vi "lijnvolgen afstandssensor.vi"() -> ()   [LabVIEW 2019]
uses:
  <vilib>/myRIO/Common/Instrument Driver Framework/Utilities/typedefs/Analog Scaling Constants.ctl
  <vilib>/myRIO/Common/Instrument Driver Framework/Utilities/typedefs/Analog Scaling Constants List.ctl
  <vilib>/myRIO/Common/Instrument Driver Framework/myRIO v1.0/AO/typedefs/AO Channels Enum.ctl
  <vilib>/myRIO/Common/Instrument Driver Framework/myRIO v1.0/AO/typedefs/AO Channels List.ctl
  <vilib>/myRIO/Common/Instrument Driver Framework/Utilities/typedefs/Generic FPGA Reference.ctl
  <vilib>/myRIO/Common/Instrument Driver Framework/Utilities/typedefs/myRIO v1.0 Reference.ctl
  <vilib>/myRIO/Common/Instrument Driver Framework/Utilities/typedefs/Hardware Version Enum.ctl
  <vilib>/myRIO/Common/Instrument Driver Framework/Utilities/typedefs/myRIO Generic Hardware Reference.ctl
  <vilib>/myRIO/Instrument Drivers/Onboard IO/AO/typedefs/AO Reference.ctl
  <vilib>/myRIO/Instrument Drivers/Onboard IO/AO/AO.lvlib
  <vilib>/myRIO/Instrument Drivers/Onboard IO/AO/vis/Write.vi
  <vilib>/userDefined/High Color/nirio_resource_hc.ctl
  <vilib>/myRIO/Common/Instrument Driver Framework/myRIO v1.0/AO/vis/myRIO v1.1 Open AO.vi
  <vilib>/myRIO/Instrument Drivers/Onboard IO/AO/vis/myRIO AO Open.xnode
  <vilib>/myRIO/Common/Instrument Driver Framework/Utilities/vis/Is FPGA Ref Available.vi
  <vilib>/myRIO/Express VI/Onboard IO/AO/AO Express VI.xnode
  <vilib>/myRIO/Common/Instrument Driver Framework/myRIO v1.0/AI/typedefs/AI Channels Enum.ctl
  <vilib>/myRIO/Common/Instrument Driver Framework/myRIO v1.0/AI/typedefs/AI Channels List.ctl
  <vilib>/myRIO/Instrument Drivers/Onboard IO/AI/typedefs/AI Reference.ctl
  <vilib>/myRIO/Instrument Drivers/Onboard IO/AI/AI.lvlib
  <vilib>/myRIO/Instrument Drivers/Onboard IO/AI/vis/Read.vi
  <vilib>/myRIO/Common/Instrument Driver Framework/myRIO v1.0/AI/vis/myRIO v1.1 Open AI.vi
  <vilib>/myRIO/Instrument Drivers/Onboard IO/AI/vis/myRIO AI Open.xnode
  <vilib>/myRIO/Express VI/Onboard IO/AI/AI Express VI.xnode
  <vilib>/myRIO/Common/Instrument Driver Framework/myRIO v1.0/DIO/typedefs/DIO Channels Enum.ctl
  <vilib>/myRIO/Common/Instrument Driver Framework/myRIO v1.0/DIO/typedefs/DIO Channels List.ctl
  <vilib>/myRIO/Instrument Drivers/Onboard IO/DIO/typedefs/DIO Reference.ctl
  <vilib>/myRIO/Instrument Drivers/Onboard IO/DIO/DIO.lvlib
  <vilib>/myRIO/Instrument Drivers/Onboard IO/DIO/vis/Read.vi
  <vilib>/myRIO/Common/Instrument Driver Framework/myRIO v1.0/DIO/vis/myRIO v1.1 Open DIO.vi
  <vilib>/myRIO/Instrument Drivers/Onboard IO/DIO/vis/myRIO DIO Open.xnode
  <vilib>/myRIO/Express VI/Onboard IO/DI/DI Express VI.xnode
panel:
  out "GEEN obstakel":bool
  in  "Hoofdwhile":bool
  out "Numeric 4":i32
  out "analoog":dbl[](array[numeric])
  out "Array 3":i32[](array[numeric])
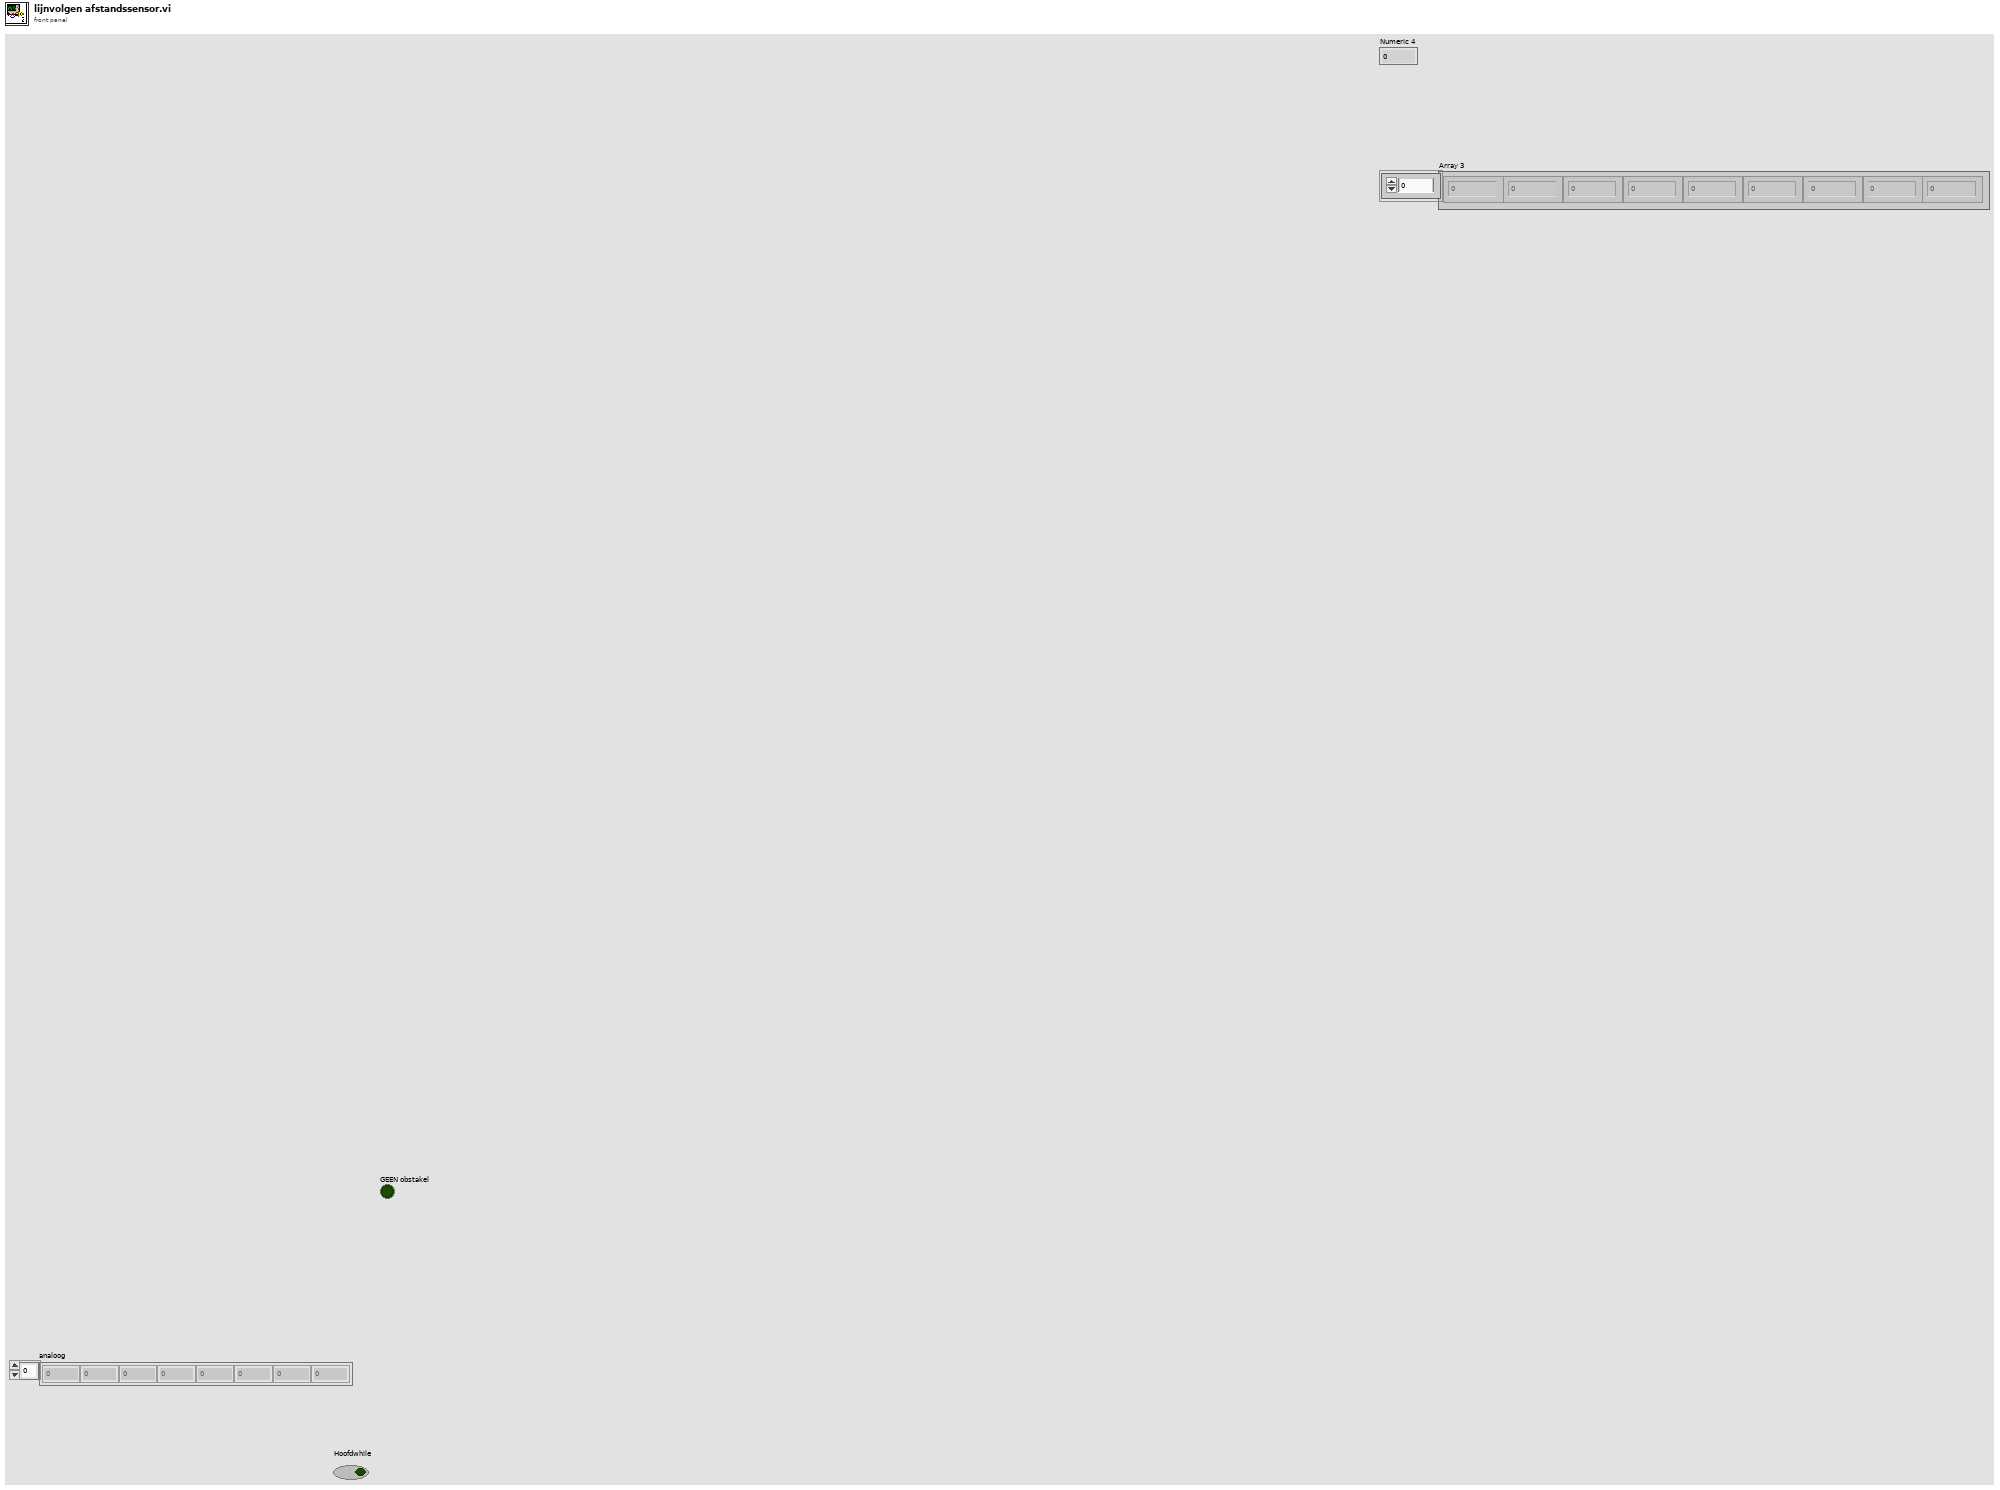
[diagram p1: front panel]
types:
  T1 = typedef "AO.lvlib/AO Reference.ctl" = cluster{"myRIO Reference":T2, "AO Channel List":T6, "AO Scaling Constant List":T8}
  T2 = typedef "myRIO Generic Hardware Reference.ctl" = cluster{"myRIO Model":T3, "myRIO Hardware Reference":T4}
  T3 = typedef "Hardware Version Enum.ctl" = enum16{"Unknown", "myRIO-1900", "myRIO-1950", "roboRIO", "NI ELVIS RIO CM", "ELVIS III"}
  T4 = typedef "myRIO v1.0 Reference.ctl" = cluster{"Generic FPGA Reference":T5, "Allow multiple opens":bool}
  T5 = typedef "Generic FPGA Reference.ctl" = refnum<k20>
  T6 = typedef "AO Channels List.ctl" = T7[]
  T7 = typedef "AO Channels Enum.ctl" = enum16{"Not Connected", "AudioOut/Left", "AudioOut/Right", "C/AO0", "C/AO1", "A/AO0", "A/AO1", "B/AO0", "B/AO1"}
  T8 = typedef "Analog Scaling Constants List.ctl" = T9[]
  T9 = typedef "Analog Scaling Constants.ctl" = cluster{"LSB Weight (Volts)":dbl, "Offset (Volts)":dbl, "Signed?":bool}
  T10 = typedef "nirio_resource_hc.ctl" = tag
  T11 = typedef "AI.lvlib/AI Reference.ctl" = cluster{"myRIO Reference":T2, "AI Channels List":T12, "AI Scaling Constants List":T8}
  T12 = typedef "AI Channels List.ctl" = T13[]
  T13 = typedef "AI Channels Enum.ctl" = enum16{"Not Connected", "AudioIn/Left", "AudioIn/Right", "C/AI0", "C/AI1", "A/AI0", "A/AI1", "A/AI2", "A/AI3", "A/AI4", "A/AI5", "A/AI6", "A/AI7", "B/AI0", "B/AI1", "B/AI2", "B/AI3", "B/AI4", "B/AI5", "B/AI6", "B/AI7", "AI/AI0", "AI/AI1", "AI/AI2", "AI/AI3", "A/AI0 (DIFF)", "A/AI1 (DIFF)", "A/AI2 (DIFF)", "A/AI3 (DIFF)", "B/AI0 (DIFF)", "B/AI1 (DIFF)", "B/AI2 (DIFF)", "B/AI3 (DIFF)"}
  T14 = typedef "DIO.lvlib/DIO Reference.ctl" = cluster{"myRIO Reference":T2, "DIO Channels List":T15}
  T15 = typedef "DIO Channels List.ctl" = T16[]
  T16 = typedef "DIO Channels Enum.ctl" = enum16{"Not Connected", "C/DIO0", "C/DIO1", "C/DIO2", "C/DIO3", "C/DIO4", "C/DIO5", "C/DIO6", "C/DIO7", "A/DIO0", "A/DIO1", "A/DIO2", "A/DIO3", "A/DIO4", "A/DIO5", "A/DIO6", "A/DIO7", "A/DIO8", "A/DIO9", "A/DIO10", "A/DIO11", "A/DIO12", "A/DIO13", "A/DIO14", "A/DIO15", "A/DIO16", "A/DIO17", "A/DIO18", "A/DIO19", "B/DIO0", "B/DIO1", "B/DIO2", "B/DIO3", "B/DIO4", "B/DIO5", "B/DIO6", "B/DIO7", "B/DIO8", "B/DIO9", "B/DIO10", "B/DIO11", "B/DIO12", "B/DIO13", "B/DIO14", "B/DIO15", "B/DIO16", "B/DIO17", "B/DIO18", "B/DIO19", "LED0", "LED1", "LED2", "LED3", "Button0", "DIO/DIO0", "DIO/DIO1", "DIO/DIO2", "DIO/DIO3", "DIO/DIO4", "DIO/DIO5", "DIO/DIO6", "DIO/DIO7", "DIO/DIO8", "DIO/DIO9", "SPI/CS0", "SPI/CS1", "SPI/CS2", "SPI/CS3", "LED RADIO (Green)", "LED RADIO (Red)", "LED COMM (Green)", "LED COMM (Red)", "LED MODE (Green)", "LED MODE (Red)"}
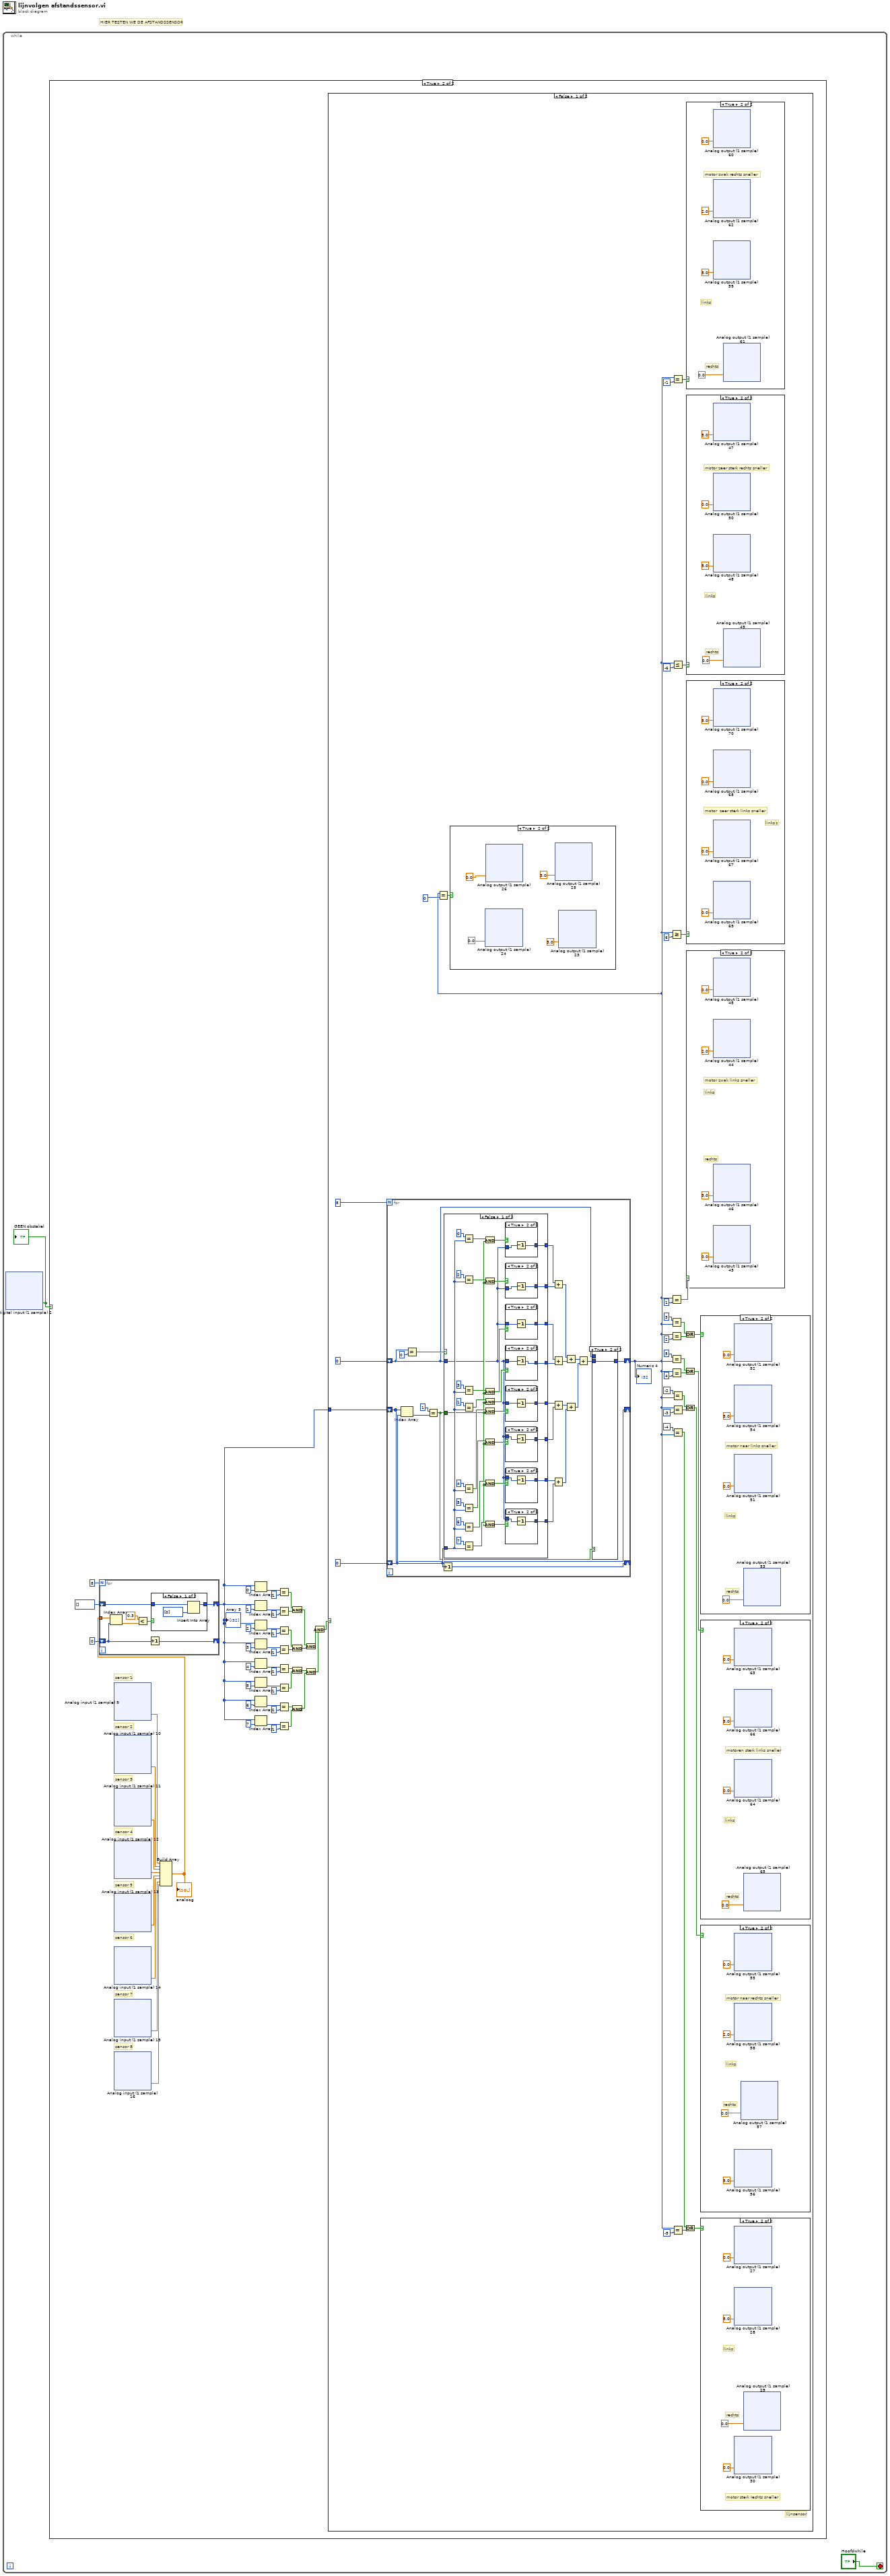
[diagram p0: block diagram]
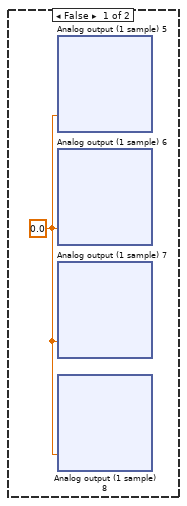
[diagram p2: hidden frame]
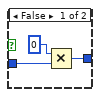
[diagram p13: hidden frame]
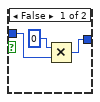
[diagram p14: hidden frame]
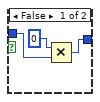
[diagram p15: hidden frame]
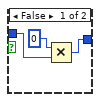
[diagram p16: hidden frame]
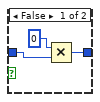
[diagram p17: hidden frame]
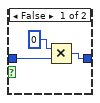
[diagram p18: hidden frame]
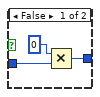
[diagram p19: hidden frame]
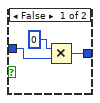
[diagram p20: hidden frame]
diagram:
  # "HIER TESTEN WE DE AFSTANDSSENSOR"
  n1 = while {
    stop <- "Hoofdwhile" stop-if-true
    n2 = xnode "Digital input (1 sample) 2"() -> ("A/DIO1 (Pin 13)"=w1:bool)  [unwired: 1 in, 1 out]
    "GEEN obstakel" <- w1
    n3 = case shown="True" w1 {
      frame False {
        w3 = 0.0
        n4 = xnode "Analog output (1 sample) 5"("A/AO0 (Pin 2)"=w3) -> ()  [unwired: 1 in, 1 out]
        n5 = xnode "Analog output (1 sample) 6"("A/AO1 (Pin 4)"=w3) -> ()  [unwired: 1 in, 1 out]
        n6 = xnode "Analog output (1 sample) 7"("B/AO0 (Pin 2)"=w3) -> ()  [unwired: 1 in, 1 out]
        n7 = xnode "Analog output (1 sample) 8"("B/AO1 (Pin 4)"=w3) -> ()  [unwired: 1 in, 1 out]
      }
      frame True {
        # "sensor 8"
        # "sensor 7"
        # "sensor 6"
        # "sensor 5"
        # "sensor 4"
        # "sensor 3"
        # "sensor 2"
        # "sensor 1"
        n8 = xnode "Analog input (1 sample) 9"() -> ("A/AI3 (Pin 9)"=w155:dbl)  [unwired: 1 in, 1 out]
        n9 = xnode "Analog input (1 sample) 10"() -> ("A/AI2 (Pin 7)"=w156:dbl)  [unwired: 1 in, 1 out]
        n10 = xnode "Analog input (1 sample) 11"() -> ("A/AI1 (Pin 5)"=w157:dbl)  [unwired: 1 in, 1 out]
        n11 = xnode "Analog input (1 sample) 12"() -> ("A/AI0 (Pin 3)"=w158:dbl)  [unwired: 1 in, 1 out]
        n12 = xnode "Analog input (1 sample) 13"() -> ("B/AI3 (Pin 9)"=w159:dbl)  [unwired: 1 in, 1 out]
        n13 = xnode "Analog input (1 sample) 14"() -> ("B/AI2 (Pin 7)"=w160:dbl)  [unwired: 1 in, 1 out]
        n14 = xnode "Analog input (1 sample) 15"() -> ("A/AI1 (Pin 5)"=w161:dbl)  [unwired: 1 in, 1 out]
        n15 = xnode "Analog input (1 sample) 16"() -> ("B/AI0 (Pin 3)"=w162:dbl)  [unwired: 1 in, 1 out]
        n16 = Build Array(w155, w156, w157, w158, w159, w160, w161, w162) -> (w154:dbl[])
        "analoog" <- w154
        n17 = for {
          N: 8 -> [_]
          shift-right: [w2244] -> w152
          shift-left: i32[] [] -> [w2245]
          shift-right: [w2241] -> _
          shift-left: 0 -> [w2240]
          tunnel: w154 -> [w2238]
          n18 = Index Array(array=w2238, index=w2240) -> (element=w2239:dbl)
          n19 = Less?(x=0.3, y=w2239) -> (x < y?=w2243:bool)
          n20 = Increment(x=w2240) -> (x+1=w2241:i32)
          n21 = case shown="False" w2243 {
            tunnel: w2245 -> [w2247 w2249]
            tunnel: [w2248 w2251] -> w2244
            frame False {
              n22 = Insert Into Array(array=w2247, new element=i32[] [0]) -> (w2248:i32[])  [unwired: 1 in]
            }
            frame True {
              n23 = Insert Into Array(array=w2249, new element=i32[] [1, 1]) -> (w2251:i32[])  [unwired: 1 in]
            }
          }
        }
        "Array 3" <- w152
        n24 = Index Array(array=w152, index=0) -> (element=w184:i32)
        n25 = Index Array(array=w152, index=1) -> (element=w163:i32)
        n26 = Index Array(array=w152, index=2) -> (element=w169:i32)
        n27 = Index Array(array=w152, index=3) -> (element=w166:i32)
        n28 = Index Array(array=w152, index=4) -> (element=w172:i32)
        n29 = Index Array(array=w152, index=5) -> (element=w175:i32)
        n30 = Index Array(array=w152, index=6) -> (element=w178:i32)
        n31 = Index Array(array=w152, index=7) -> (element=w181:i32)
        n32 = Equal?(x=w184, y=1) -> (x = y?=w187:bool)
        n33 = Equal?(x=w163, y=1) -> (x = y?=w188:bool)
        n34 = Equal?(x=w169, y=1) -> (x = y?=w189:bool)
        n35 = Equal?(x=w166, y=1) -> (x = y?=w190:bool)
        n36 = Equal?(x=w172, y=1) -> (x = y?=w191:bool)
        n37 = Equal?(x=w175, y=1) -> (x = y?=w192:bool)
        n38 = Equal?(x=w178, y=1) -> (x = y?=w193:bool)
        n39 = Equal?(x=w181, y=1) -> (x = y?=w194:bool)
        n40 = And(x=w187, y=w188) -> (x .and. y?=w195:bool)
        n41 = And(x=w189, y=w190) -> (x .and. y?=w196:bool)
        n42 = And(x=w191, y=w192) -> (x .and. y?=w197:bool)
        n43 = And(x=w193, y=w194) -> (x .and. y?=w198:bool)
        n44 = And(x=w195, y=w196) -> (x .and. y?=w199:bool)
        n45 = And(x=w197, y=w198) -> (x .and. y?=w200:bool)
        n46 = And(x=w199, y=w200) -> (x .and. y?=w153:bool)
        n47 = case shown="False" w153 {
          tunnel: w152 -> [w204 _]
          frame False {
            # "lijnsensor"
            n48 = for {
              N: 8 -> [_]
              shift-right: [w1617] -> _
              shift-left: 0 -> [w1631]
              shift-right: [w1609] -> w205
              shift-left: 0 -> [w1610]
              shift-right: [w1622] -> _
              shift-left: w204 -> [w1622]
              n49 = Index Array(array=w1622, index=w1631) -> (element=w1621:i32)
              n50 = Equal?(x=w1610, y=0) -> (x = y?=w1618:bool)
              n51 = Equal?(x=1, y=w1621) -> (x = y?=w1608:bool)
              n52 = Increment(x=w1631) -> (x+1=w1617:i32)
              n53 = case shown="False" w1618 {
                tunnel: w1631 -> [w1641 w1727]
                tunnel: [w1635 w1726] -> w1630
                tunnel: [w1642 w1725] -> w1629
                tunnel: [w1643 w1724] -> w1628
                tunnel: [w1644 w1723] -> w1627
                tunnel: w1610 -> [w1634 w1722]
                tunnel: w1608 -> [w1640 w1713]
                tunnel: [w1638 w1712] -> w1616
                tunnel: [w1639 w1711] -> w1615
                tunnel: [w1636 w1710] -> w1613
                tunnel: [w1637 w1709] -> w1612
                frame False {
                  n54 = Equal?(x=0, y=w1641) -> (x = y?=w1661:bool)
                  n55 = Equal?(x=2, y=w1641) -> (x = y?=w1667:bool)
                  n56 = Equal?(x=3, y=w1641) -> (x = y?=w1668:bool)
                  n57 = Equal?(x=1, y=w1641) -> (x = y?=w1653:bool)
                  n58 = Equal?(x=4, y=w1641) -> (x = y?=w1665:bool)
                  n59 = Equal?(x=5, y=w1641) -> (x = y?=w1666:bool)
                  n60 = Equal?(x=6, y=w1641) -> (x = y?=w1664:bool)
                  n61 = Equal?(x=7, y=w1641) -> (x = y?=w1663:bool)
                  n62 = And(x=w1661, y=w1640) -> (x .and. y?=w1645:bool)
                  n63 = And(x=w1667, y=w1640) -> (x .and. y?=w1647:bool)
                  n64 = And(x=w1668, y=w1640) -> (x .and. y?=w1648:bool)
                  n65 = And(x=w1653, y=w1640) -> (x .and. y?=w1646:bool)
                  n66 = And(x=w1665, y=w1640) -> (x .and. y?=w1649:bool)
                  n67 = And(x=w1666, y=w1640) -> (x .and. y?=w1650:bool)
                  n68 = And(x=w1664, y=w1640) -> (x .and. y?=w1651:bool)
                  n69 = And(x=w1663, y=w1640) -> (x .and. y?=w1652:bool)
                  n70 = case shown="True" w1645 {
                    tunnel: [w1670 w1673] -> w1639
                    tunnel: w1634 -> [w1669 w1672]
                    frame False {
                      n71 = Multiply(x=0, y=w1669) -> (x*y=w1670:i32)
                    }
                    frame True {
                      n72 = Decrement(x=w1672) -> (x-1=w1673:i32)
                    }
                  }
                  n73 = case shown="True" w1647 {
                    tunnel: [w1701 w1702] -> w1638
                    tunnel: w1634 -> [w1700 w1703]
                    frame False {
                      n74 = Multiply(x=0, y=w1700) -> (x*y=w1701:i32)
                    }
                    frame True {
                      n75 = Decrement(x=w1703) -> (x-1=w1702:i32)
                    }
                  }
                  n76 = case shown="True" w1648 {
                    tunnel: [w1695 w1698] -> w1637
                    tunnel: w1634 -> [w1694 w1697]
                    frame False {
                      n77 = Multiply(x=0, y=w1694) -> (x*y=w1695:i32)
                    }
                    frame True {
                      n78 = Decrement(x=w1697) -> (x-1=w1698:i32)
                    }
                  }
                  n79 = case shown="True" w1646 {
                    tunnel: [w1705 w1708] -> w1636
                    tunnel: w1634 -> [w1704 w1707]
                    frame False {
                      n80 = Multiply(x=0, y=w1704) -> (x*y=w1705:i32)
                    }
                    frame True {
                      n81 = Decrement(x=w1707) -> (x-1=w1708:i32)
                    }
                  }
                  n82 = case shown="True" w1649 {
                    tunnel: [w1690 w1693] -> w1635
                    tunnel: w1634 -> [w1689 w1692]
                    frame False {
                      n83 = Multiply(x=0, y=w1689) -> (x*y=w1690:i32)
                    }
                    frame True {
                      n84 = Decrement(x=w1692) -> (x-1=w1693:i32)
                    }
                  }
                  n85 = case shown="True" w1650 {
                    tunnel: [w1680 w1683] -> w1642
                    tunnel: w1634 -> [w1679 w1682]
                    frame False {
                      n86 = Multiply(x=0, y=w1679) -> (x*y=w1680:i32)
                    }
                    frame True {
                      n87 = Decrement(x=w1682) -> (x-1=w1683:i32)
                    }
                  }
                  n88 = case shown="True" w1651 {
                    tunnel: [w1685 w1688] -> w1643
                    tunnel: w1634 -> [w1684 w1687]
                    frame False {
                      n89 = Multiply(x=0, y=w1684) -> (x*y=w1685:i32)
                    }
                    frame True {
                      n90 = Decrement(x=w1687) -> (x-1=w1688:i32)
                    }
                  }
                  n91 = case shown="True" w1652 {
                    tunnel: [w1674 w1678] -> w1644
                    tunnel: w1634 -> [w1675 w1677]
                    frame False {
                      n92 = Multiply(x=0, y=w1675) -> (x*y=w1674:i32)
                    }
                    frame True {
                      n93 = Decrement(x=w1677) -> (x-1=w1678:i32)
                    }
                  }
                }
                frame True {
                  n94 = Equal?(x=0, y=w1727) -> (x = y?=w1736:bool)
                  n95 = Equal?(x=1, y=w1727) -> (x = y?=w1728:bool)
                  n96 = Equal?(x=2, y=w1727) -> (x = y?=w1742:bool)
                  n97 = Equal?(x=3, y=w1727) -> (x = y?=w1743:bool)
                  n98 = Equal?(x=4, y=w1727) -> (x = y?=w1740:bool)
                  n99 = Equal?(x=5, y=w1727) -> (x = y?=w1741:bool)
                  n100 = Equal?(x=6, y=w1727) -> (x = y?=w1739:bool)
                  n101 = Equal?(x=7, y=w1727) -> (x = y?=w1738:bool)
                  n102 = And(x=w1736, y=w1713) -> (x .and. y?=w1714:bool)
                  n103 = And(x=w1728, y=w1713) -> (x .and. y?=w1715:bool)
                  n104 = And(x=w1742, y=w1713) -> (x .and. y?=w1716:bool)
                  n105 = And(x=w1743, y=w1713) -> (x .and. y?=w1717:bool)
                  n106 = And(x=w1740, y=w1713) -> (x .and. y?=w1718:bool)
                  n107 = And(x=w1741, y=w1713) -> (x .and. y?=w1719:bool)
                  n108 = And(x=w1739, y=w1713) -> (x .and. y?=w1720:bool)
                  n109 = And(x=w1738, y=w1713) -> (x .and. y?=w1721:bool)
                  n110 = case shown="True" w1714 {
                    tunnel: w1722 -> [w1744 w1748]
                    tunnel: [w1745 w1747] -> w1711
                    frame False {
                      n111 = Multiply(x=0, y=w1744) -> (x*y=w1745:i32)
                    }
                    frame True {
                      n112 = Add(x=7, y=w1748) -> (x+y=w1747:i32)
                    }
                  }
                  n113 = case shown="True" w1715 {
                    tunnel: w1722 -> [w1784 w1787]
                    tunnel: [w1785 w1788] -> w1712
                    frame False {
                      n114 = Multiply(x=0, y=w1784) -> (x*y=w1785:i32)
                    }
                    frame True {
                      n115 = Add(x=5, y=w1787) -> (x+y=w1788:i32)
                    }
                  }
                  n116 = case shown="True" w1716 {
                    tunnel: w1722 -> [w1778 w1782]
                    tunnel: [w1779 w1781] -> w1709
                    frame False {
                      n117 = Multiply(x=0, y=w1778) -> (x*y=w1779:i32)
                    }
                    frame True {
                      n118 = Add(x=3, y=w1782) -> (x+y=w1781:i32)
                    }
                  }
                  n119 = case shown="True" w1717 {
                    tunnel: w1722 -> [w1774 w1777]
                    tunnel: [w1773 w1776] -> w1710
                    frame False {
                      n120 = Multiply(x=0, y=w1774) -> (x*y=w1773:i32)
                    }
                    frame True {
                      n121 = Increment(x=w1777) -> (x+1=w1776:i32)
                    }
                  }
                  n122 = case shown="True" w1718 {
                    tunnel: w1722 -> [w1768 w1772]
                    tunnel: [w1769 w1771] -> w1726
                    frame False {
                      n123 = Multiply(x=0, y=w1768) -> (x*y=w1769:i32)
                    }
                    frame True {
                      n124 = Decrement(x=w1772) -> (x-1=w1771:i32)
                    }
                  }
                  n125 = case shown="True" w1719 {
                    tunnel: w1722 -> [w1757 w1759]
                    tunnel: [w1756 w1761] -> w1725
                    frame False {
                      n126 = Multiply(x=0, y=w1757) -> (x*y=w1756:i32)
                    }
                    frame True {
                      n127 = Subtract(x=w1759, y=3) -> (x-y=w1761:i32)
                    }
                  }
                  n128 = case shown="True" w1720 {
                    tunnel: w1722 -> [w1763 w1765]
                    tunnel: [w1762 w1766] -> w1724
                    frame False {
                      n129 = Multiply(x=0, y=w1763) -> (x*y=w1762:i32)
                    }
                    frame True {
                      n130 = Subtract(x=w1765, y=5) -> (x-y=w1766:i32)
                    }
                  }
                  n131 = case shown="True" w1721 {
                    tunnel: w1722 -> [w1750 w1753]
                    tunnel: [w1751 w1754] -> w1723
                    frame False {
                      n132 = Multiply(x=0, y=w1750) -> (x*y=w1751:i32)
                    }
                    frame True {
                      n133 = Subtract(x=w1753, y=7) -> (x-y=w1754:i32)
                    }
                  }
                }
              }
              n134 = Add(x=w1615, y=w1616) -> (x+y=w1614:i32)
              n135 = Add(x=w1612, y=w1613) -> (x+y=w1611:i32)
              n136 = Add(x=w1630, y=w1629) -> (x+y=w1625:i32)
              n137 = Add(x=w1628, y=w1627) -> (x+y=w1626:i32)
              n138 = Add(x=w1614, y=w1611) -> (x+y=w1624:i32)
              n139 = Add(x=w1625, y=w1626) -> (x+y=w1623:i32)
              n140 = Add(x=w1624, y=w1623) -> (x+y=w1607:i32)
              n141 = case shown="True" w1608 {
                tunnel: w1610 -> [w1632 _]
                tunnel: [w1632 w1633] -> w1609
                tunnel: w1607 -> [_ w1633]
                frame False {
                }
                frame True {
                }
              }
            }
            "Numeric 4" <- w205
            n142 = Equal?(x=w205, y=0) -> (x = y?=w207:bool)
            n143 = case shown="True" w207 {
              frame False {
              }
              frame True {
                n144 = xnode "Analog output (1 sample) 24"("B/AO0 (Pin 2)"=0.0) -> ()  [unwired: 1 in, 1 out]
                n145 = xnode "Analog output (1 sample) 26"("A/AO0 (Pin 2)"=0.0) -> ()  [unwired: 1 in, 1 out]
                n146 = xnode "Analog output (1 sample) 25"("A/AO1 (Pin 4)"=3.0) -> ()  [unwired: 1 in, 1 out]
                n147 = xnode "Analog output (1 sample) 23"("B/AO1 (Pin 4)"=3.0) -> ()  [unwired: 1 in, 1 out]
              }
            }
            n148 = Greater Or Equal?(x=w205, y=6) -> (x >= y?=w233:bool)
            n149 = Equal?(x=w205, y=1) -> (x = y?=w234:bool)
            n150 = Equal?(x=3, y=w205) -> (x = y?=w224:bool)
            n151 = Equal?(x=w205, y=2) -> (x = y?=w225:bool)
            n152 = Equal?(x=5, y=w205) -> (x = y?=w228:bool)
            n153 = Equal?(x=w205, y=4) -> (x = y?=w229:bool)
            n154 = Equal?(x=w205, y=-1) -> (x = y?=w212:bool)
            n155 = Less Or Equal?(x=w205, y=-6) -> (x <= y?=w210:bool)
            n156 = Equal?(x=-2, y=w205) -> (x = y?=w218:bool)
            n157 = Equal?(x=w205, y=-3) -> (x = y?=w219:bool)
            n158 = Equal?(x=-4, y=w205) -> (x = y?=w214:bool)
            n159 = Equal?(x=w205, y=-5) -> (x = y?=w215:bool)
            n160 = Or(x=w224, y=w225) -> (x .or. y?=w222:bool)
            n161 = Or(x=w228, y=w229) -> (x .or. y?=w230:bool)
            n162 = Or(x=w218, y=w219) -> (x .or. y?=w211:bool)
            n163 = Or(x=w214, y=w215) -> (x .or. y?=w208:bool)
            n164 = case shown="True" w212 {
              frame False {
              }
              frame True {
                # "rechts"
                # "links"
                # "motor zwak rechts sneller"
                n165 = xnode "Analog output (1 sample) 60"("B/AO1 (Pin 4)"=0.0) -> ()  [unwired: 1 in, 1 out]
                n166 = xnode "Analog output (1 sample) 62"("A/AO0 (Pin 2)"=2.0) -> ()  [unwired: 1 in, 1 out]
                n167 = xnode "Analog output (1 sample) 59"("B/AO0 (Pin 2)"=5.0) -> ()  [unwired: 1 in, 1 out]
                n168 = xnode "Analog output (1 sample) 61"("A/AO1 (Pin 4)"=0.0) -> ()  [unwired: 1 in, 1 out]
              }
            }
            n169 = case shown="True" w210 {
              frame False {
              }
              frame True {
                # "rechts"
                # "links"
                # "motor zeer sterk rechts sneller"
                n170 = xnode "Analog output (1 sample) 47"("B/AO1 (Pin 4)"=5.0) -> ()  [unwired: 1 in, 1 out]
                n171 = xnode "Analog output (1 sample) 50"("A/AO0 (Pin 2)"=0.0) -> ()  [unwired: 1 in, 1 out]
                n172 = xnode "Analog output (1 sample) 48"("B/AO0 (Pin 2)"=5.0) -> ()  [unwired: 1 in, 1 out]
                n173 = xnode "Analog output (1 sample) 49"("A/AO1 (Pin 4)"=0.0) -> ()  [unwired: 1 in, 1 out]
              }
            }
            n174 = case shown="True" w233 {
              frame False {
              }
              frame True {
                # "rechts"
                # "links"
                # "motor  zeer sterk links sneller"
                n175 = xnode "Analog output (1 sample) 70"("A/AO0 (Pin 2)"=5.0) -> ()  [unwired: 1 in, 1 out]
                n176 = xnode "Analog output (1 sample) 68"("B/AO0 (Pin 2)"=0.0) -> ()  [unwired: 1 in, 1 out]
                n177 = xnode "Analog output (1 sample) 67"("B/AO1 (Pin 4)"=0.0) -> ()  [unwired: 1 in, 1 out]
                n178 = xnode "Analog output (1 sample) 69"("A/AO1 (Pin 4)"=0.0) -> ()  [unwired: 1 in, 1 out]
              }
            }
            n179 = case shown="True" w234 {
              frame False {
              }
              frame True {
                # "rechts"
                # "links"
                # "motor zwak links sneller"
                n180 = xnode "Analog output (1 sample) 45"("A/AO1 (Pin 4)"=0.0) -> ()  [unwired: 1 in, 1 out]
                n181 = xnode "Analog output (1 sample) 44"("B/AO0 (Pin 2)"=2.0) -> ()  [unwired: 1 in, 1 out]
                n182 = xnode "Analog output (1 sample) 46"("A/AO0 (Pin 2)"=5.0) -> ()  [unwired: 1 in, 1 out]
                n183 = xnode "Analog output (1 sample) 43"("B/AO1 (Pin 4)"=0.0) -> ()  [unwired: 1 in, 1 out]
              }
            }
            n184 = case shown="True" w222 {
              frame False {
              }
              frame True {
                # "rechts"
                # "links"
                # "motor naar links sneller"
                n185 = xnode "Analog output (1 sample) 52"("B/AO0 (Pin 2)"=0.0) -> ()  [unwired: 1 in, 1 out]
                n186 = xnode "Analog output (1 sample) 54"("A/AO0 (Pin 2)"=5.0) -> ()  [unwired: 1 in, 1 out]
                n187 = xnode "Analog output (1 sample) 51"("B/AO1 (Pin 4)"=0.0) -> ()  [unwired: 1 in, 1 out]
                n188 = xnode "Analog output (1 sample) 53"("A/AO1 (Pin 4)"=0.0) -> ()  [unwired: 1 in, 1 out]
              }
            }
            n189 = case shown="True" w230 {
              frame False {
              }
              frame True {
                # "rechts"
                # "links"
                # "motoren sterk links sneller"
                n190 = xnode "Analog output (1 sample) 63"("B/AO1 (Pin 4)"=0.0) -> ()  [unwired: 1 in, 1 out]
                n191 = xnode "Analog output (1 sample) 66"("A/AO0 (Pin 2)"=5.0) -> ()  [unwired: 1 in, 1 out]
                n192 = xnode "Analog output (1 sample) 64"("B/AO0 (Pin 2)"=0.0) -> ()  [unwired: 1 in, 1 out]
                n193 = xnode "Analog output (1 sample) 65"("A/AO1 (Pin 4)"=0.0) -> ()  [unwired: 1 in, 1 out]
              }
            }
            n194 = case shown="True" w211 {
              frame False {
              }
              frame True {
                # "rechts"
                # "links"
                # "motor naar rechts sneller"
                n195 = xnode "Analog output (1 sample) 55"("B/AO1 (Pin 4)"=0.0) -> ()  [unwired: 1 in, 1 out]
                n196 = xnode "Analog output (1 sample) 58"("A/AO0 (Pin 2)"=2.0) -> ()  [unwired: 1 in, 1 out]
                n197 = xnode "Analog output (1 sample) 56"("B/AO0 (Pin 2)"=5.0) -> ()  [unwired: 1 in, 1 out]
                n198 = xnode "Analog output (1 sample) 57"("A/AO1 (Pin 4)"=0.0) -> ()  [unwired: 1 in, 1 out]
              }
            }
            n199 = case shown="True" w208 {
              frame False {
              }
              frame True {
                # "rechts"
                # "links"
                # "motor sterk rechts sneller"
                n200 = xnode "Analog output (1 sample) 27"("B/AO1 (Pin 4)"=0.0) -> ()  [unwired: 1 in, 1 out]
                n201 = xnode "Analog output (1 sample) 28"("B/AO0 (Pin 2)"=5.0) -> ()  [unwired: 1 in, 1 out]
                n202 = xnode "Analog output (1 sample) 30"("A/AO0 (Pin 2)"=0.0) -> ()  [unwired: 1 in, 1 out]
                n203 = xnode "Analog output (1 sample) 29"("A/AO1 (Pin 4)"=0.0) -> ()  [unwired: 1 in, 1 out]
              }
            }
          }
          frame True {
            n204 = xnode "Analog output (1 sample)"("A/AO0 (Pin 2)"=0) -> ()  [unwired: 1 in, 1 out]
            n205 = xnode "Analog output (1 sample) 3"("B/AO0 (Pin 2)"=0) -> ()  [unwired: 1 in, 1 out]
            n206 = xnode "Analog output (1 sample) 2"("A/AO1 (Pin 4)"=0) -> ()  [unwired: 1 in, 1 out]
            n207 = xnode "Analog output (1 sample) 4"("B/AO1 (Pin 4)"=0) -> ()  [unwired: 1 in, 1 out]
          }
        }
      }
    }
  }
